vi "u2uw.vi"(2 "error in (no error)":errorcluster, 3 "u":dbl) -> (0 "error out":errorcluster, 1 "uw":dbl)   [LabVIEW 2021]
panel:
  out "In Range?":bool
  out "Vin":dbl
  out "J":dbl
  out "CD":dbl
  out "b":dbl
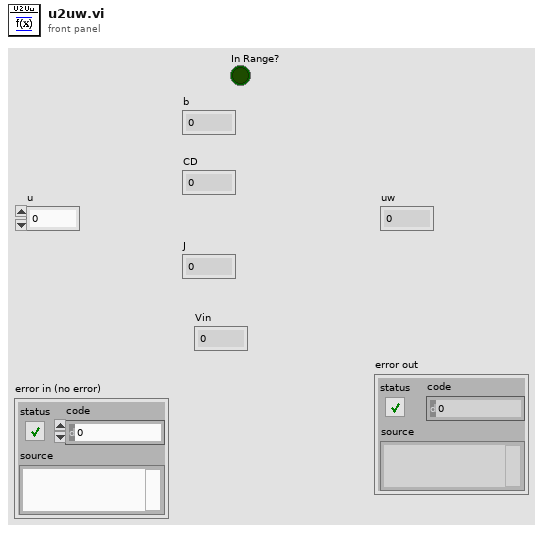
[diagram p1: front panel]
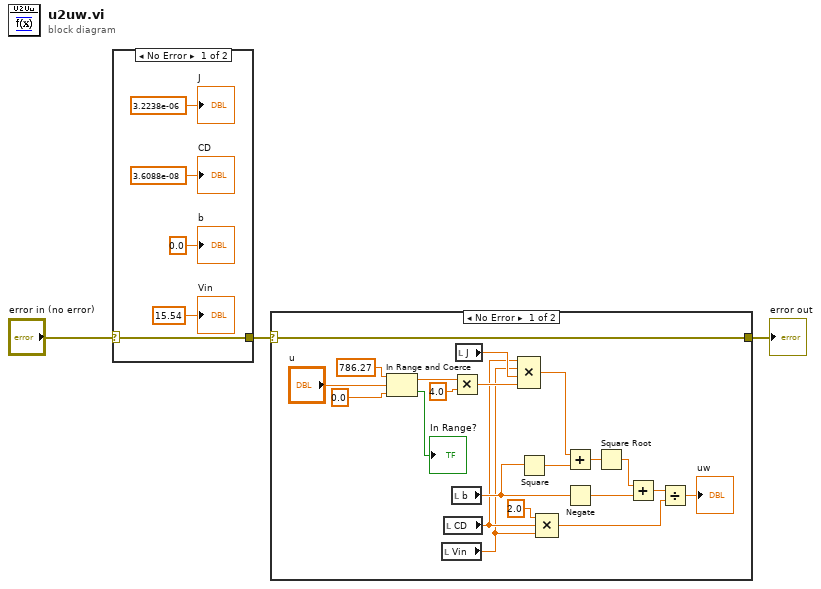
[diagram p0: block diagram]
diagram:
  n1 = case shown="No Error" "error in (no error)" {
    selector: "error in (no error)" -> [w4 w9]
    tunnel: [w4 w9] -> w2
    frame No Error {
      "b" <- 0.0 ("b")
      "CD" <- 3.6088e-08 ("CD")
      "J" <- 3.2238e-06 ("J")
      "Vin" <- 15.54 ("Vin")
    }
    frame Error {
    }
  }
  n2 = case shown="No Error" w2 {
    selector: w2 -> [w30 w31]
    tunnel: [w30 w31] -> w1
    frame No Error {
      n3 = In Range and Coerce(upper limit=786.27, x="u", lower limit=0.0) -> (coerced(x)=w14:dbl, In Range?=→"In Range?":bool)
      n4 = local read "Vin"() -> (w16:dbl)
      n5 = local read "CD"() -> (w17:dbl)
      n6 = Multiply(x=w14, y=4.0) -> (x*y=w27:dbl)
      n7 = local read "b"() -> (w21:dbl)
      n8 = local read "J"() -> (w28:dbl)
      n9 = Compound Arithmetic op=MULTIPLY(w17, w16, w28, w27) -> (w26:dbl)
      n10 = Square(x=w21) -> (x^2=w25:dbl)
      n11 = Compound Arithmetic op=MULTIPLY(2.0 ("value"), w17, w16) -> (w19:dbl)
      n12 = Add(x=w26, y=w25) -> (x+y=w24:dbl)
      n13 = Negate(x=w21) -> (-x=w22:dbl)
      n14 = Square Root(x=w24) -> (sqrt(x)=w23:dbl)
      n15 = Add(x=w23, y=w22) -> (x+y=w20:dbl)
      n16 = Divide(x=w20, y=w19) -> (x/y=→"uw":dbl)
    }
    frame Error {
    }
  }
  "error out" <- w1
